vi "toXml.vi"(8 "error in (no error)":errorcluster, 11 "rf in":refnum<class "rf.lvclass">) -> (0 "error out":errorcluster, 2 "scriptEventXML":refnum<class "xmlNode.lvclass">, 3 "rf out":refnum<class "rf.lvclass">)   [LabVIEW 2011, in "Tools.lvlib" / "Scripting.lvlib" / "rf.lvclass"]
uses:
  rf.lvclass
  xmlNode/xmlNode.lvclass
  ScriptEvent.lvclass
  DatabaseHelpers/Database Objects/Channel/Channel.lvclass
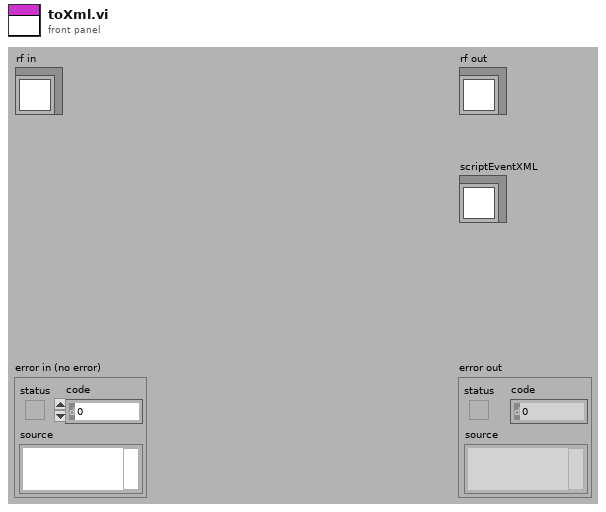
[diagram p1: front panel]
types:
  T1 = cluster{"attributeName":string, "channel_name":string}
  T2 = cluster{"attributeName":string, "channel_name":string}[]
  T3 = cluster{"parameter_name":string, "parameter_value":string, "type":enum16{"time", "time_difference", "value", "frequency", "phase", "ramp_time", "value_step", "time_step", "number_of_steps", "start_value", "end_value", "start_freq", "start_amp", "start_phase", "end_freq", "end_amp", "end_phase"}}[]
  T4 = enum16{"time", "time_difference", "value", "frequency", "phase", "ramp_time", "value_step", "time_step", "number_of_steps", "start_value", "end_value", "start_freq", "start_amp", "start_phase", "end_freq", "end_amp", "end_phase"}
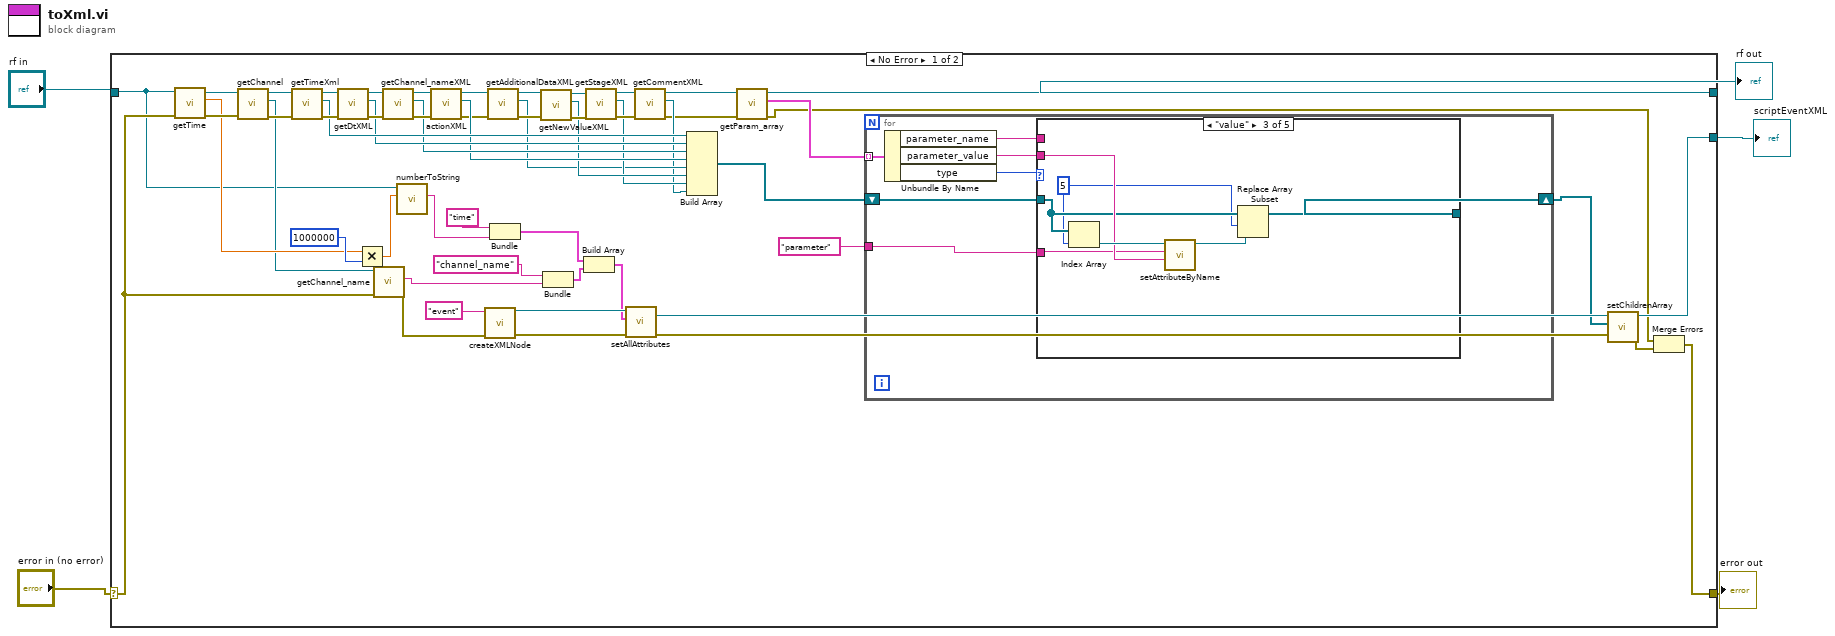
[diagram p0: block diagram]
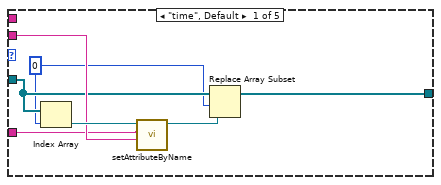
[diagram p2: hidden frame]
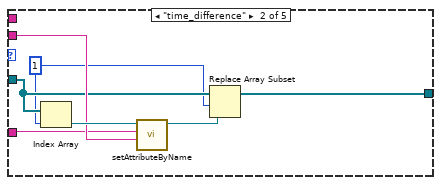
[diagram p3: hidden frame]
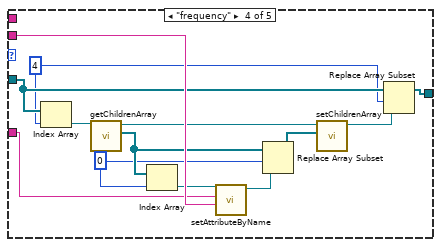
[diagram p4: hidden frame]
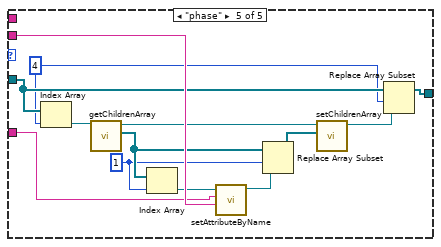
[diagram p5: hidden frame]
diagram:
  n1 = case shown="No Error" "error in (no error)" {
    selector: "error in (no error)" -> [w25 w117]
    tunnel: "rf in" -> [w17 w116]
    tunnel: [w13 w116] -> w4
    tunnel: [w24 w117] -> w3
    tunnel: [w7 _] -> w1
    frame No Error {
      n2 = call "getTime.vi"("error in (no error)"=w25, "ScriptEvent.lvclass in"=w17) -> ("error out"=w30:errorcluster, "time"=w27:dbl, "ScriptEvent.lvclass out"=w28:refnum<class "rf.lvclass">)  [unwired: 7 in]
      n3 = call-dynamic "getChannel.vi"("error in (no error)"=w30, "ScriptEvent.lvclass in"=w28) -> ("error out"=w31:errorcluster, "Channel.lvclass"=w26:refnum<class "Channel.lvclass">, "ScriptEvent.lvclass out"=w29:refnum<class "rf.lvclass">)  [unwired: 7 in]
      n4 = call "getTimeXml.vi"("error in (no error)"=w31, "ScriptEvent in"=w29) -> ("error out"=w59:errorcluster, "timeXML"=w49:refnum<class "xmlNode.lvclass">, "ScriptEvent out"=w54:refnum<class "rf.lvclass">)  [unwired: 7 in]
      n5 = call "getDtXML.vi"("error in (no error)"=w59, "ScriptEvent in"=w54) -> ("error out"=w58:errorcluster, "dtXML"=w48:refnum<class "xmlNode.lvclass">, "ScriptEvent out"=w53:refnum<class "rf.lvclass">)  [unwired: 7 in]
      n6 = Multiply(x=w27, y=1000000) -> (x*y=w16:dbl)
      n7 = call "getChannel_name.vi"("error in (no error)"=w25, "Channel.lvclass in"=w26) -> ("error out"=w60:errorcluster, "channel_name"=w40:string)  [unwired: 7 in, 1 out]
      n8 = call "getChannel_nameXML.vi"("error in (no error)"=w58, "ScriptEvent in"=w53) -> ("error out"=w57:errorcluster, "channel_nameXML"=w47:refnum<class "xmlNode.lvclass">, "ScriptEvent out"=w52:refnum<class "rf.lvclass">)  [unwired: 7 in]
      n9 = call "numberToString.vi"("Numeric"=w16, "ScriptEvent in"=w17) -> ("String"=w15:string)  [unwired: 7 in, 2 out]
      n10 = call "actionXML.vi"("error in (no error)"=w57, "ScriptEvent in"=w52) -> ("error out"=w21:errorcluster, "actionXml"=w46:refnum<class "xmlNode.lvclass">, "ScriptEvent out"=w23:refnum<class "rf.lvclass">)  [unwired: 7 in]
      n11 = call "createXMLNode.vi"("error in (no error)"=w60, "name"="event") -> ("error out"=w35:errorcluster, "xmlNode out"=w39:refnum<class "xmlNode.lvclass">)  [unwired: 8 in]
      n12 = call-dynamic "getAdditionalDataXML.vi"("error in (no error)"=w21, "rf in"=w23) -> ("error out"=w20:errorcluster, "additionalDataXML"=w19:refnum<class "xmlNode.lvclass">, "rf out"=w22:refnum<class "rf.lvclass">)  [unwired: 7 in]
      n13 = Bundle("attributeName"="time", "String"=w15) -> (w38:cluster{"attributeName":string, "String":string})  [unwired: 1 in]
      n14 = call-dynamic "getNewValueXML.vi"("error in (no error)"=w20, "ScriptEvent in"=w22) -> ("error out"=w56:errorcluster, "newValueXML"=w45:refnum<class "xmlNode.lvclass">, "ScriptEvent out"=w51:refnum<class "rf.lvclass">)  [unwired: 7 in]
      n15 = Bundle("attributeName"="channel_name", "channel_name"=w40) -> (w37:T1)  [unwired: 1 in]
      n16 = Build Array(w38, w37) -> (w36:T2)
      n17 = call "getStageXML.vi"("error in (no error)"=w56, "ScriptEvent in"=w51) -> ("error out"=w55:errorcluster, "stageXML"=w44:refnum<class "xmlNode.lvclass">, "ScriptEvent out"=w50:refnum<class "rf.lvclass">)  [unwired: 7 in]
      n18 = call-dynamic "setAllAttributes.vi"("error in (no error)"=w35, "attributes"=w36, "xmlNode in"=w39) -> ("error out"=w34:errorcluster, "xmlNode out"=w33:refnum<class "xmlNode.lvclass">)  [unwired: 7 in]
      n19 = call "getCommentXML.vi"("error in (no error)"=w55, "ScriptEvent in"=w50) -> ("error out"=w10:errorcluster, "commentXML"=w18:refnum<class "xmlNode.lvclass">, "ScriptEvent out"=w14:refnum<class "rf.lvclass">)  [unwired: 7 in]
      n20 = Build Array(w49, w48, w47, w46, w19, w45, w44, w18) -> (w11:refnum<class "xmlNode.lvclass">[])
      n21 = call "getParam_array.vi"("error in (no error)"=w10, "ScriptEvent in"=w14) -> ("error out"=w6:errorcluster, "param_array"=w12:T3, "ScriptEvent out"=w13:refnum<class "rf.lvclass">)  [unwired: 7 in]
      n22 = for {
        shift-right: [w64] -> w8
        shift-left: w11 -> [w67]
        tunnel: w12 -> [w63] mode=indexing
        tunnel: "parameter" -> [w62]
        n23 = Unbundle By Name(w63) -> ("parameter_name"=w66:string, "parameter_value"=w65:string, "type"=w68:T4)
        n24 = case shown="\"value\"" w68 {
          tunnel: w67 -> [w72 w79 w86 w101 w114]
          tunnel: w66 -> [_ _ _ _ _]
          tunnel: w65 -> [w74 w81 w88 w102 w115]
          tunnel: [w70 w77 w84 w99 w112] -> w64
          tunnel: w62 -> [w69 w76 w83 w90 w103]
          frame "time", Default {
            w71 = 0
            n25 = Index Array(array=w72, index=w71) -> (element=w75:refnum<class "xmlNode.lvclass">)
            n26 = call-dynamic "setAttributeByName.vi"("attributeValue"=w74, "attributeName"=w69, "xmlNode in"=w75) -> ("xmlNode out"=w73:refnum<class "xmlNode.lvclass">)  [unwired: 7 in, 1 out]
            n27 = Replace Array Subset(array=w72, new element=w73, index=w71) -> (w70:refnum<class "xmlNode.lvclass">[])
          }
          frame "time_difference" {
            w78 = 1
            n28 = Index Array(array=w79, index=w78) -> (element=w82:refnum<class "xmlNode.lvclass">)
            n29 = call-dynamic "setAttributeByName.vi"("attributeValue"=w81, "attributeName"=w76, "xmlNode in"=w82) -> ("xmlNode out"=w80:refnum<class "xmlNode.lvclass">)  [unwired: 7 in, 1 out]
            n30 = Replace Array Subset(array=w79, new element=w80, index=w78) -> (w77:refnum<class "xmlNode.lvclass">[])
          }
          frame "value" {
            w85 = 5
            n31 = Index Array(array=w86, index=w85) -> (element=w89:refnum<class "xmlNode.lvclass">)
            n32 = call-dynamic "setAttributeByName.vi"("attributeValue"=w88, "attributeName"=w83, "xmlNode in"=w89) -> ("xmlNode out"=w87:refnum<class "xmlNode.lvclass">)  [unwired: 7 in, 1 out]
            n33 = Replace Array Subset(array=w86, new element=w87, index=w85) -> (w84:refnum<class "xmlNode.lvclass">[])
          }
          frame "frequency" {
            w91 = 0
            w100 = 4
            n34 = Index Array(array=w101, index=w100) -> (element=w98:refnum<class "xmlNode.lvclass">)
            n35 = call-dynamic "getChildrenArray.vi"("xmlNode.lvclass in"=w98) -> ("Children"=w96:refnum<class "xmlNode.lvclass">[], "xmlNode.lvclass out"=w94:refnum<class "xmlNode.lvclass">)  [unwired: 8 in, 1 out]
            n36 = Index Array(array=w96, index=w91) -> (element=w97:refnum<class "xmlNode.lvclass">)
            n37 = call-dynamic "setAttributeByName.vi"("attributeValue"=w102, "attributeName"=w90, "xmlNode in"=w97) -> ("xmlNode out"=w95:refnum<class "xmlNode.lvclass">)  [unwired: 7 in, 1 out]
            n38 = Replace Array Subset(array=w96, new element=w95, index=w91) -> (w93:refnum<class "xmlNode.lvclass">[])
            n39 = call-dynamic "setChildrenArray.vi"("Children"=w93, "xmlNode.lvclass in"=w94) -> ("xmlNode.lvclass out"=w92:refnum<class "xmlNode.lvclass">)  [unwired: 8 in, 1 out]
            n40 = Replace Array Subset(array=w101, new element=w92, index=w100) -> (w99:refnum<class "xmlNode.lvclass">[])
          }
          frame "phase" {
            w104 = 1
            w113 = 4
            n41 = Index Array(array=w114, index=w113) -> (element=w111:refnum<class "xmlNode.lvclass">)
            n42 = call-dynamic "getChildrenArray.vi"("xmlNode.lvclass in"=w111) -> ("Children"=w109:refnum<class "xmlNode.lvclass">[], "xmlNode.lvclass out"=w107:refnum<class "xmlNode.lvclass">)  [unwired: 8 in, 1 out]
            n43 = Index Array(array=w109, index=w104) -> (element=w110:refnum<class "xmlNode.lvclass">)
            n44 = call-dynamic "setAttributeByName.vi"("attributeValue"=w115, "attributeName"=w103, "xmlNode in"=w110) -> ("xmlNode out"=w108:refnum<class "xmlNode.lvclass">)  [unwired: 7 in, 1 out]
            n45 = Replace Array Subset(array=w109, new element=w108, index=w104) -> (w106:refnum<class "xmlNode.lvclass">[])
            n46 = call-dynamic "setChildrenArray.vi"("Children"=w106, "xmlNode.lvclass in"=w107) -> ("xmlNode.lvclass out"=w105:refnum<class "xmlNode.lvclass">)  [unwired: 8 in, 1 out]
            n47 = Replace Array Subset(array=w114, new element=w105, index=w113) -> (w112:refnum<class "xmlNode.lvclass">[])
          }
        }
      }
      n48 = call-dynamic "setChildrenArray.vi"("error in (no error)"=w34, "Children"=w8, "xmlNode.lvclass in"=w33) -> ("error out"=w43:errorcluster, "xmlNode.lvclass out"=w7:refnum<class "xmlNode.lvclass">)  [unwired: 7 in]
      n49 = Merge Errors(w6, w43) -> (w24:errorcluster)
    }
    frame Error {
    }
  }
  "error out" <- w3
  "rf out" <- w4
  "scriptEventXML" <- w1
